vi "Check_Reading.vi"(1 "Saving File Path":path) -> (0 "data":string[][](array[string]))   [LabVIEW 2020]
uses:
  <vilib>/Utility/NIReport.llb/Report Type.ctl
  <vilib>/express/express shared/transition.llb/Dynamic To Waveform Array.vi
  <vilib>/express/express signal manip/GetorSetDDTAttributes/Set DDT Attributes/SetT0.vi
  <vilib>/express/express shared/transition.llb/Waveform Array To Dynamic.vi
  <vilib>/addons/_office/excel.llb/Excel Get Data ([str]).vi
  <vilib>/express/express signal manip/GetorSetDDTAttributes/Set DDT Attributes/Set DDT Properties.xnode
  <vilib>/Utility/NIReport.llb/NI_report.lvclass
  <vilib>/Utility/NIReport.llb/Excel/NI_Excel.lvclass
  <vilib>/Utility/NIReport.llb/NI_ReportGenerationCore.lvlib
  <vilib>/addons/_office/NI_ReportGenerationToolkit.lvlib
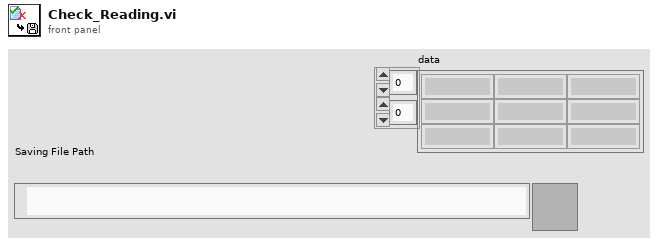
[diagram p1: front panel]
types:
  T1 = typedef "NI_ReportGenerationCore.lvlib/Report Type.ctl" = enum16{"HTML", "Word", "Excel"}
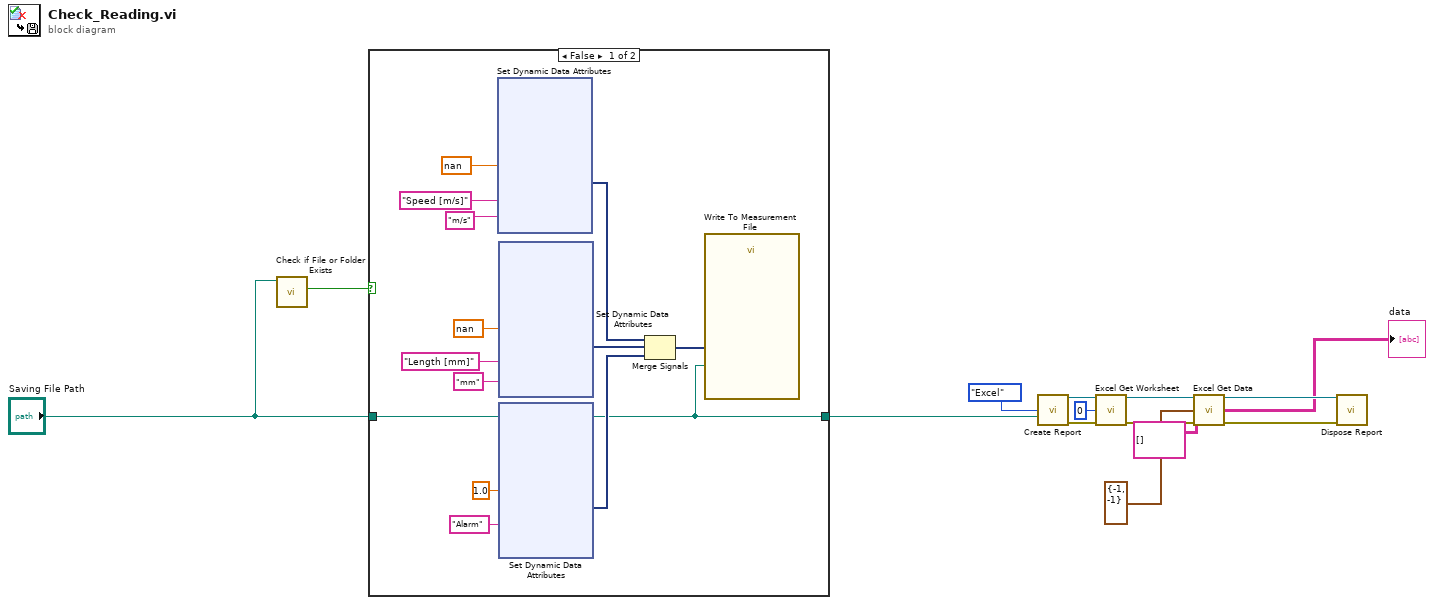
[diagram p0: block diagram]
diagram:
  n1 = call <vilib>:"Check if File or Folder Exists.vi"("path"="Saving File Path") -> ("file or folder exists?"=w2:bool)  [unwired: 8 in, 2 out]
  n2 = case shown="False" w2 {
    tunnel: [w17 w82] -> w3
    tunnel: "Saving File Path" -> [w17 w82]
    frame False {
      n3 = xnode "Set Dynamic Data Attributes"("Signals In"=nan, "Signal Name"="Speed [m/s]", "Unit"="m/s") -> ("Signals Out"=w23:dynamicdata)  [unwired: 2 in, 1 out]
      n4 = xnode "Set Dynamic Data Attributes"("Signals In"=nan, "Signal Name"="Length [mm]", "Unit"="mm") -> ("Signals Out"=w22:dynamicdata)  [unwired: 2 in, 1 out]
      n5 = xnode "Set Dynamic Data Attributes"("Signals In"=1.0, "Signal Name"="Alarm") -> ("Signals Out"=w21:dynamicdata)  [unwired: 3 in, 1 out]
      n6 = Merge Signals(w23, w22, w21) -> (w20:dynamicdata)
      n7 = call "Write To Measurement File"("Signals"=w20, "Filename"=w17) -> ()  [unwired: 15 in, 3 out]
    }
    frame True {
    }
  }
  n8 = call <vilib>:"Create Report.vi"("report type"=Report_Type."Excel", "template (empty)"=w3) -> ("report out"=w12:refnum<class "NI_report.lvclass">, "error out"=w13:errorcluster)  [unwired: 12 in]
  n9 = call <vilib>:"Excel Get Worksheet.vi"("report in"=w12, "worksheet index (0)"=0, "error in (no error)"=w13) -> ("report out"=w10:refnum<class "NI_report.lvclass">, "error out"=w9:errorcluster)  [unwired: 11 in]
  n10 = call-poly <vilib>:"Excel Get Data.vi"("report in"=w10, "data type"=string[][] [], "start (-1, -1)"=cluster{"start row":i32, "start column":i32} {"start row"=-1, "start column"=-1} ("start (0, 0)"), "error in (no error)"=w9) -> ("report out"=w6:refnum<class "NI_report.lvclass">, "data"=→"data":string[][], "error out"=w5:errorcluster)  [unwired: 9 in]
  n11 = call-dynamic "Dispose Report.vi"("report in"=w6, "error in (no error)"=w5) -> ()  [unwired: 13 in, 1 out]
